vi "Scope Names.vi"(10 "Type Name":string, 11 "Container Name":string) -> (3 "Scope Names":string[](array[string]))   [LabVIEW 2020, in "LV-Protoc.lvlib" / "LV-Protoc.lvclass"]
uses:
  LV-Protoc.lvclass
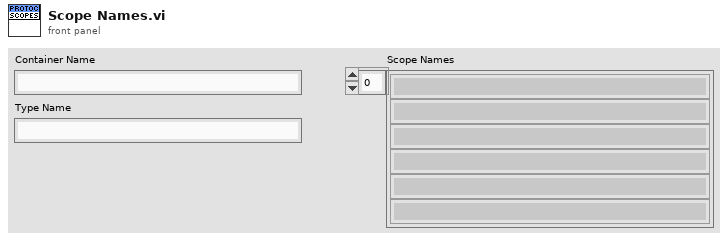
[diagram p1: front panel]
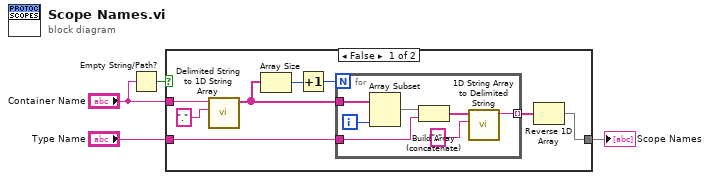
[diagram p0: block diagram]
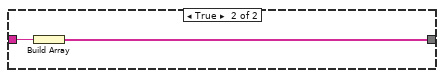
[diagram p2: hidden frame]
diagram:
  n1 = Empty String/Path?(string/path="Container Name") -> (empty?=w4:bool)
  n2 = case shown="False" w4 {
    tunnel: "Container Name" -> [w12 _]
    tunnel: "Type Name" -> [w9 w21]
    tunnel: [w5 w20] -> w1
    frame False {
      n3 = call <vilib>:"Delimited String to 1D String Array.vi"("delimiter"=".", "delimited string"=w12) -> ("string array"=w8:string[])  [unwired: 9 in]
      n4 = Array Size(array=w8) -> (size(s)=w7:i32)
      n5 = Increment(x=w7) -> (x+1=w6:i32)
      n6 = for {
        N: w6 -> [_]
        tunnel: w9 -> [w16]
        tunnel: w8 -> [w19]
        tunnel: [w13] -> w10 mode=indexing
        i -> [w18]
        n7 = Array Subset(array=w19, length=w18) -> (w17:string[])  [unwired: 1 in]
        n8 = Build Array (concatenate)(w17, w16) -> (w15:string[])
        n9 = call <vilib>:"1D String Array to Delimited String.vi"("delimiter"=".", "string array"=w15) -> ("delimited string"=w13:string)  [unwired: 9 in]
      }
      n10 = Reverse 1D Array(array=w10) -> (reversed array=w5:string[])
    }
    frame True {
      n11 = Build Array(w21) -> (w20:string[])
    }
  }
  "Scope Names" <- w1
